vi "acquireAmscopeReference.vi"() -> (3 "objRef":dbl[][](graph))   [LabVIEW 2012]
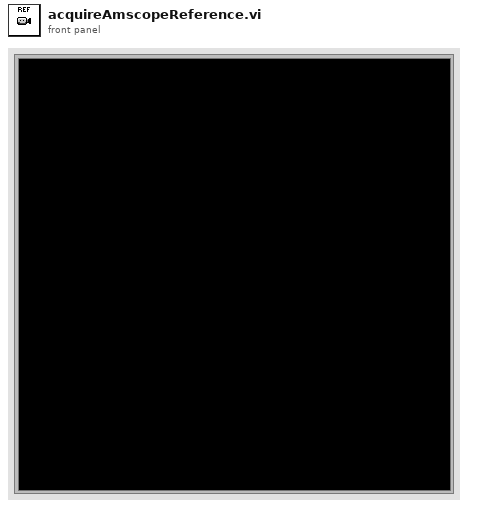
[diagram p1: front panel]
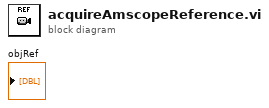
[diagram p0: block diagram]
diagram:
